vi "ErrorHandling.Fglb.Clear.vi"(7 "Event source":T1, 8 "error in (no error)":errorcluster) -> (0 "error out":errorcluster)   [LabVIEW 2016]
uses:
  EventLog/EventLog.EventSource.ctl
  ErrorHandling.Fglb.Action.ctl
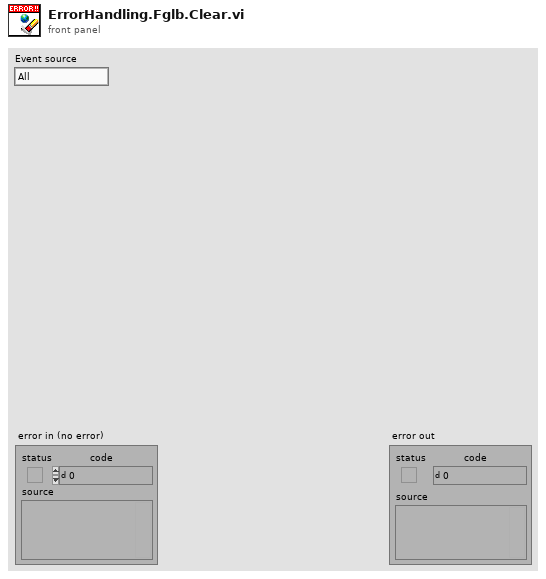
[diagram p1: front panel]
types:
  T1 = typedef "EventLog.EventSource.ctl" = enum16{"All", "Gui", "Ref", "File", "Arch", "Seq", "CPX", "DB", "Laser", "Scan.P", "Scan.O"}
  T2 = typedef "ErrorHandling.Fglb.Action.ctl" = enum16{"init", "add", "clear", "confirm", "check", "get"}
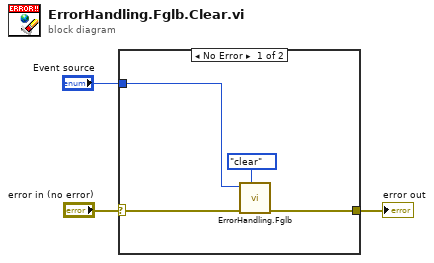
[diagram p0: block diagram]
diagram:
  n1 = case shown="No Error" "error in (no error)" {
    selector: "error in (no error)" -> [w5 w8]
    tunnel: [w6 w8] -> w3
    tunnel: "Event source" -> [w4 _]
    frame No Error {
      n2 = call "ErrorHandling.Fglb.vi"("Action"=ErrorHandling.Fglb.Action."clear", "error in (no error)"=w5, "Event source"=w4) -> ("error out"=w6:errorcluster)  [unwired: 6 in, 2 out]
    }
    frame Error {
    }
  }
  "error out" <- w3
